vi "Read Layout.vi"(8 "error in (no error)":errorcluster, 11 "ProjectBase in":refnum<class "Project.lvclass">) -> (0 "error out":errorcluster, 2 "Layout":T1={"Order"=enum."LeftRight", "Row"=2, "Column"=2, "Margin"=5}, 3 "ProjectBase out":refnum<class "Project.lvclass">)   [LabVIEW 2015, in "Project.lvclass"]
uses:
  Project.lvclass
  Project.lvclass/Project.ctl
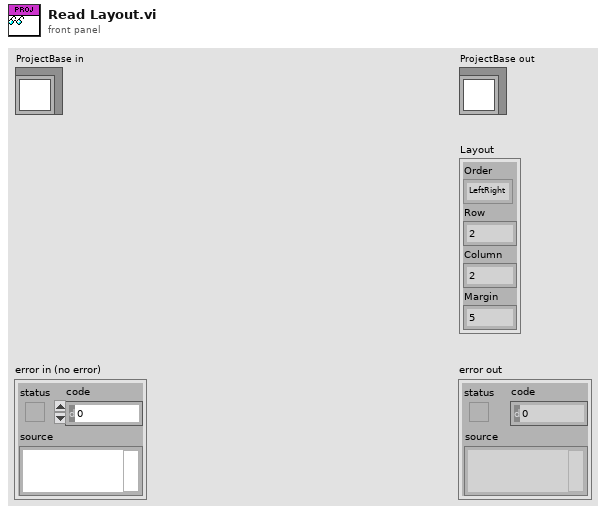
[diagram p1: front panel]
types:
  T1 = cluster{"Order":enum16{"LeftRight", "TopDown"}, "Row":i32, "Column":i32, "Margin":i32}
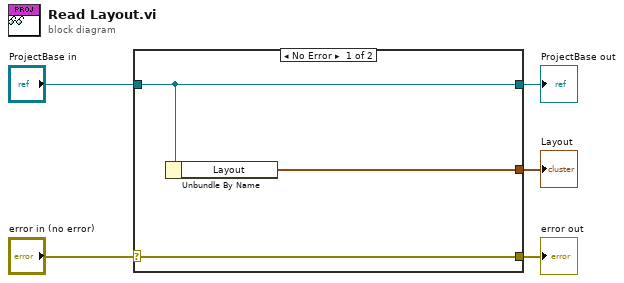
[diagram p0: block diagram]
diagram:
  n1 = case shown="No Error" "error in (no error)" {
    selector: "error in (no error)" -> [w8 w9]
    tunnel: [w8 w9] -> w4
    tunnel: [w7 w10] -> w2
    tunnel: "ProjectBase in" -> [w7 w10]
    tunnel: [w6 _] -> w1
    frame No Error {
      n2 = Unbundle By Name(w7) -> ("Layout"=w6:T1)
    }
    frame Error {
    }
  }
  "error out" <- w4
  "ProjectBase out" <- w2
  "Layout" <- w1
